vi "Send Message.vi"(4 "error in (no error)":errorcluster, 5 "Message":variant, 6 "Event":string, 7 "Queue in":refnum<queue>) -> (0 "error out":errorcluster, 3 "Queue out":refnum<queue>)   [LabVIEW 2020, in "QHM.lvlib"]
uses:
  QHM.lvlib
  Type Defs/QMH Cluster.ctl
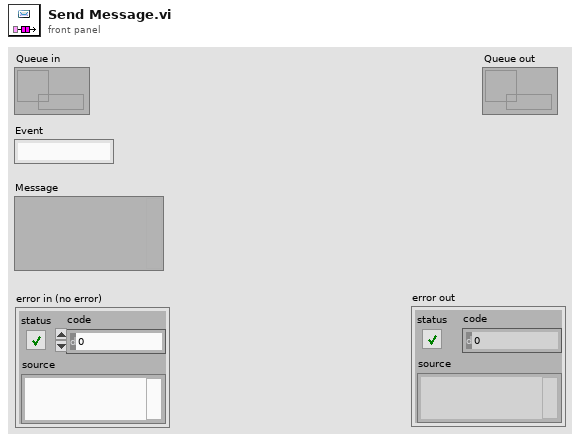
[diagram p1: front panel]
types:
  T1 = typedef "QHM.lvlib/QMH Cluster.ctl" = cluster{"Event":string, "Message":variant}
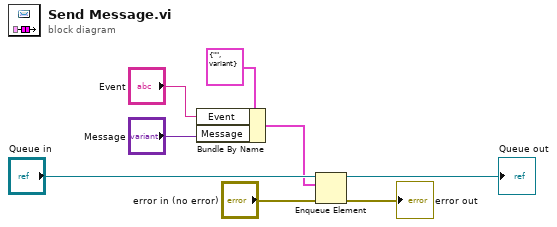
[diagram p0: block diagram]
diagram:
  n1 = Bundle By Name(cluster=T1 {"Event"="", "Message"=variant}, "Event"="Event", "Message"="Message") -> (w6:T1)
  n2 = Enqueue Element(queue="Queue in", element=w6, error in (no error)="error in (no error)") -> (queue out=→"Queue out":refnum<queue>, error out=→"error out":errorcluster)  [unwired: 1 in, 1 out]
